vi "ConvertTextBasedCodeToLabVIEW_ChangeInterfaceToInheritace.vi"(8 "error in (no error)":errorcluster, 10 "InterfacesThatShouldBeConvertedToClasses":string[](array[string]), 11 "ClassesIn":T1[](array[typedef])) -> (0 "error out":errorcluster, 3 "ClassesOut":T1[](array[typedef]))   [LabVIEW 2014]
uses:
  <resource>/Framework/Providers/Open_GDS/ClassProviders/Common/String/GDSString_ClassDescriptionType.ctl
  <resource>/Framework/Providers/Open_GDS/ClassProviders/Common/String/GDSString_AccessScopeModifierType.ctl
  <resource>/Framework/Providers/Open_GDS/ClassProviders/Common/String/GDSString_ModifierType.ctl
  <resource>/Framework/Providers/Open_GDS/ClassProviders/Common/String/GDSString_MethodDescriptionType.ctl
  <resource>/Framework/Providers/Open_GDS/ClassProviders/Common/CommonVIs/CommonVIs_AttributeType.ctl
  <resource>/Framework/Providers/Open_GDS/ClassProviders/Common/CommonVIs/CommonVIs_AttributeDataType.ctl
  <resource>/Framework/Providers/Open_GDS/ClassProviders/Common/CommonVIs/CommonVIs_PropertyType.ctl
  <resource>/Framework/Providers/Open_GDS/ClassProviders/Common/String/GDSString_ClassParentType.ctl
  <resource>/Framework/Providers/Open_GDS/ClassProviders/Common/String/GDSString_ClassType.ctl
  <resource>/Framework/Providers/Open_GDS/ClassProviders/Common/String/GDSString_ClassOwnerType.ctl
  <resource>/Framework/Providers/Open_GDS/ClassProviders/Common/CommonVIs/CommonVIs_EnumType.ctl
  <resource>/Framework/Providers/Open_GDS/ClassProviders/Common/CommonVIs/CommonVIs_StructType.ctl
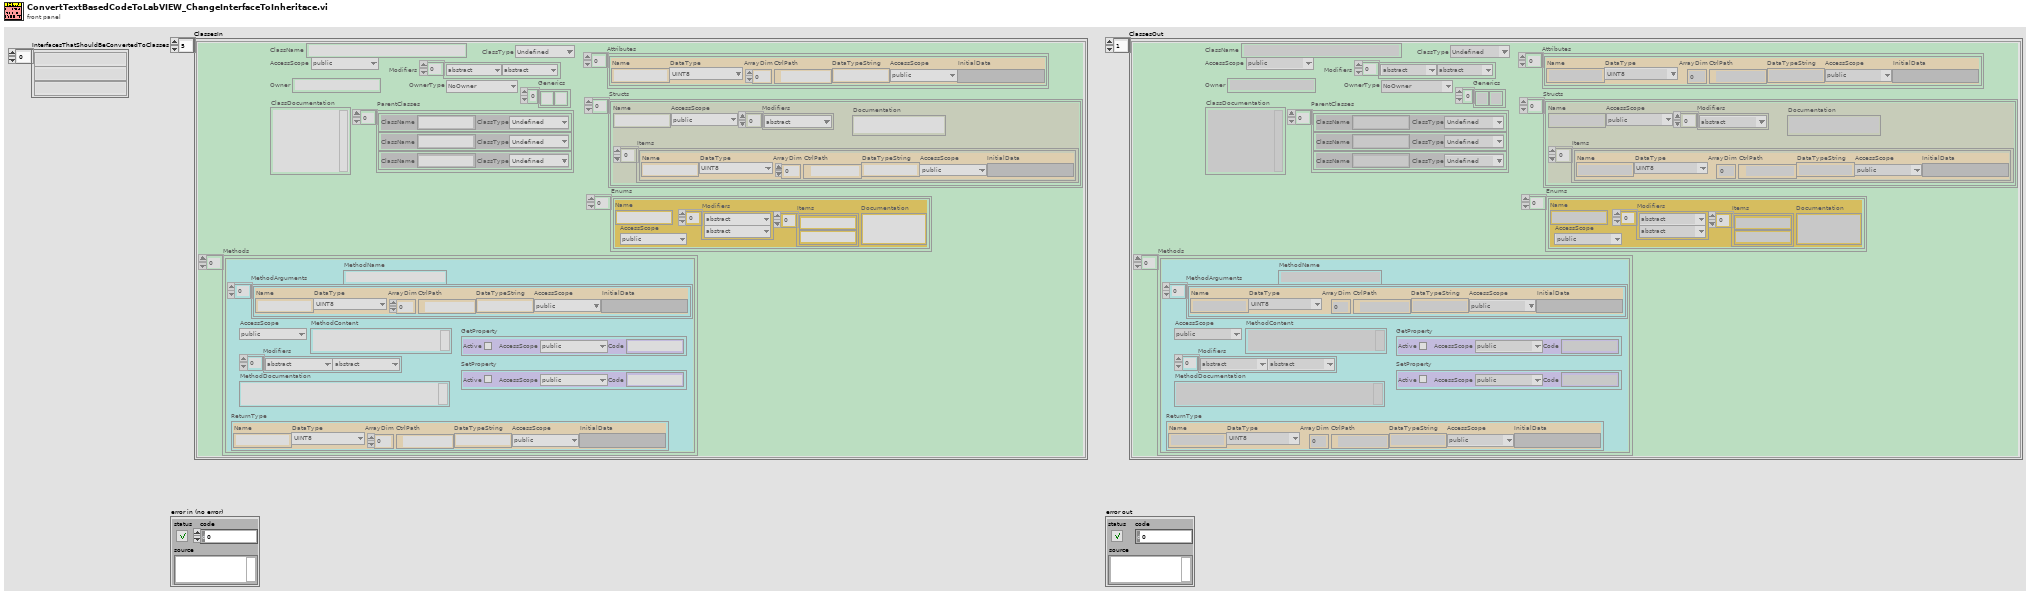
[diagram p1: front panel]
types:
  T1 = typedef "GDSString_ClassDescriptionType.ctl" = cluster{"ClassName":string, "AccessScope":T2, "Modifiers":T3[], "ClassDocumentation":string, "Methods":T4[], "ParentClasses":T8[], "ClassType":T9, "Owner":string, "OwnerType":T10, "Generics":string[], "Attributes":T5[], "Enums":T11[], "Structs":T12[]}
  T2 = typedef "GDSString_AccessScopeModifierType.ctl" = enum16{"public", "private", "protected", "internal"}
  T3 = typedef "GDSString_ModifierType.ctl" = enum16{"abstract", "static", "final", "synchronized", "strictfp", "async", "const", "event", "extern", "new", "native ", "override", "partial", "readonly", "sealed", "unsafe", "virtual", "volatile"}
  T4 = typedef "GDSString_MethodDescriptionType.ctl" = cluster{"ReturnType":T5, "MethodName":string, "AccessScope":T2, "Modifiers":T3[], "MethodDocumentation":string, "MethodContent":string, "MethodArguments":T5[], "GetProperty":T7, "SetProperty":T7}
  T5 = typedef "CommonVIs_AttributeType.ctl" = cluster{"Name":string, "DataType":T6, "ArrayDim":i32, "CtrlPath":path, "DataTypeString":string, "AccessScope":T2, "InitialData":variant}
  T6 = typedef "CommonVIs_AttributeDataType.ctl" = enum16{"UINT8", "INT8", "UINT16", "INT16", "UINT32", "INT32", "UINT64", "INT64", "SGL", "DBL", "EXT", "CSG", "CDB", "CXT", "TimeStamp", "STRING", "PATH", "BOOL", "ENUM", "RefNum", "VIRefNum", "LabVIEW Class", "Cluster", "Variant", "TypeDef", "Waveform", "LabVIEW Object", "Other", "void"}
  T7 = typedef "CommonVIs_PropertyType.ctl" = cluster{"Active":bool, "AccessScope":T2, "Code":string}
  T8 = typedef "GDSString_ClassParentType.ctl" = cluster{"ClassName":string, "ClassType":T9}
  T9 = typedef "GDSString_ClassType.ctl" = enum16{"Undefined", "Class", "Interface"}
  T10 = typedef "GDSString_ClassOwnerType.ctl" = enum16{"NoOwner", "Class", "Package/NameSpace"}
  T11 = typedef "CommonVIs_EnumType.ctl" = cluster{"Name":string, "AccessScope":T2, "Modifiers":T3[], "Items":string[], "Documentation":string}
  T12 = typedef "CommonVIs_StructType.ctl" = cluster{"Name":string, "AccessScope":T2, "Modifiers":T3[], "Items":T5[], "Documentation":string}
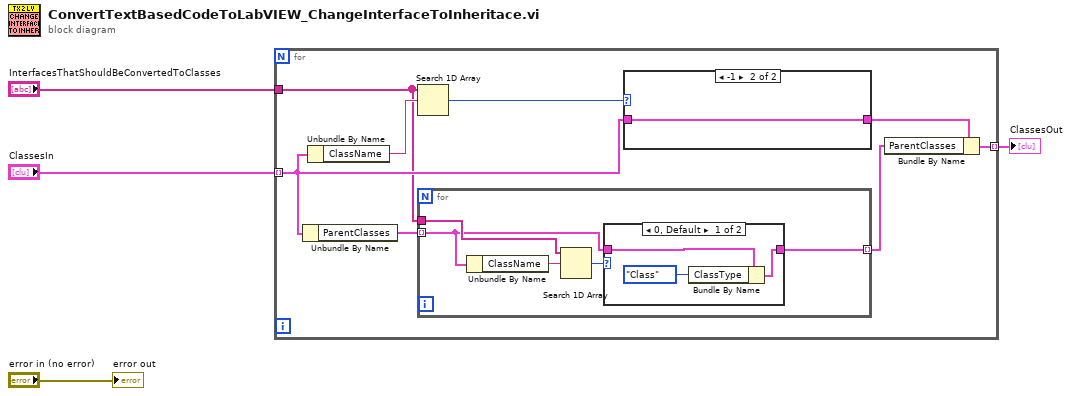
[diagram p0: block diagram]
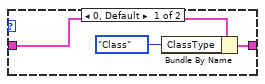
[diagram p3: hidden frame]
diagram:
  n1 = for {
    tunnel: "ClassesIn" -> [w10] mode=indexing
    tunnel: "InterfacesThatShouldBeConvertedToClasses" -> [w8]
    tunnel: [w6] -> w1 mode=indexing
    n2 = Unbundle By Name(w10) -> ("ParentClasses"=w9:T8[])
    n3 = Unbundle By Name(w10) -> ("ClassName"=w12:string)
    n4 = Search 1D Array(1D array=w8, element=w12) -> (index of element=w11:i32)  [unwired: 1 in]
    n5 = for {
      tunnel: w9 -> [w14] mode=indexing
      tunnel: w8 -> [w16]
      tunnel: [w13] -> w5 mode=indexing
      n6 = Unbundle By Name(w14) -> ("ClassName"=w17:string)
      n7 = Search 1D Array(1D array=w16, element=w17) -> (index of element=w15:i32)  [unwired: 1 in]
      n8 = case shown="0, Default" w15 {
        tunnel: w14 -> [w20 w21]
        tunnel: [w19 w21] -> w13
        frame 0, Default {
          n9 = Bundle By Name(cluster=w20, "ClassType"=GDSString_ClassType."Class") -> (w19:T8)
        }
        frame -1 {
        }
      }
    }
    n10 = case shown="-1" w11 {
      tunnel: w10 -> [w24 w25]
      tunnel: [w23 w25] -> w7
      frame 0, Default {
        n11 = Bundle By Name(cluster=w24, "ClassType"=GDSString_ClassType."Class") -> (w23:T1)
      }
      frame -1 {
      }
    }
    n12 = Bundle By Name(cluster=w7, "ParentClasses"=w5) -> (w6:T1)
  }
  "ClassesOut" <- w1
  "error out" <- "error in (no error)"
